vi "FP_Show Hide Items.vi"(8 "Error":errorcluster, 9 "FP Show Hide":T1, 11 "VI":refnum<vi>) -> (0 "Error Out":errorcluster, 3 "VI Out":refnum<vi>)   [LabVIEW 2025]
uses:
  TypeDefs_Utility/Cluster_FP_Show Hide Items.ctl
  TypeDefs_Utility/ENUM_FP_Show-Hide Select.ctl
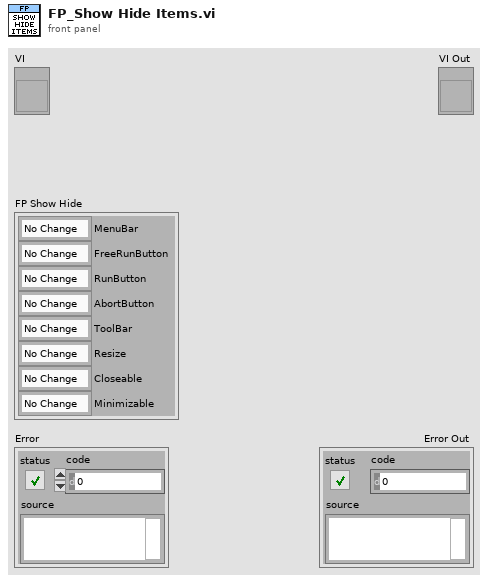
[diagram p1: front panel]
types:
  T1 = typedef "Cluster_FP_Show Hide Items.ctl" = cluster{"MenuBar":T2, "FreeRunButton":T2, "RunButton":T2, "AbortButton":T2, "ToolBar":T2, "Resize":T2, "Closeable":T2, "Minimizable":T2}
  T2 = typedef "ENUM_FP_Show-Hide Select.ctl" = enum16{"No Change", "Hide", "Show"}
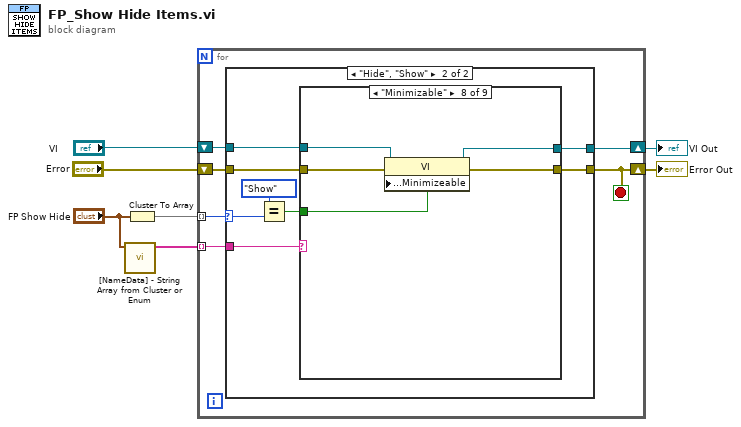
[diagram p0: block diagram]
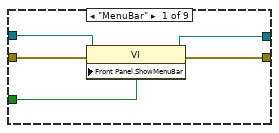
[diagram p3: hidden frame]
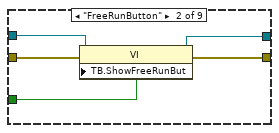
[diagram p4: hidden frame]
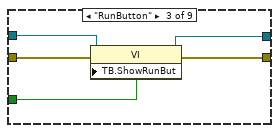
[diagram p5: hidden frame]
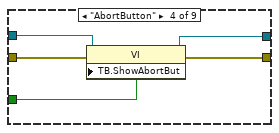
[diagram p6: hidden frame]
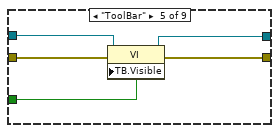
[diagram p7: hidden frame]
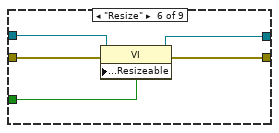
[diagram p8: hidden frame]
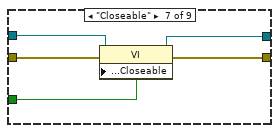
[diagram p9: hidden frame]
diagram:
  n1 = call "[NameData] - String Array from Cluster or Enum.vi"("Enum or\nCluster"="FP Show Hide") -> ("Name Array Out"=w1:string[])  [unwired: 8 in, 2 out]
  n2 = Cluster To Array(cluster="FP Show Hide") -> (array=w2:T2[])
  n3 = for {
    shift-right: [w13] -> w6
    shift-left: "VI" -> [w12]
    shift-right: [w8] -> w7
    shift-left: "Error" -> [w11]
    tunnel: w2 -> [w9] mode=indexing
    tunnel: w1 -> [w10] mode=indexing
    stop <- w8 stop-if-true
    n4 = case shown="\"Hide\", \"Show\"" w9 {
      selector: w9 -> [_ w18]
      tunnel: [w15 w23] -> w13
      tunnel: w12 -> [w15 w22]
      tunnel: w11 -> [w14 w21]
      tunnel: [w14 w20] -> w8
      tunnel: w10 -> [_ w19]
      frame "No Change" {
      }
      frame "Hide", "Show" {
        n5 = Equal?(x=ENUM_FP_Show-Hide_Select."Show" ("y"), y=w18) -> (x = y?=w16:bool)
        n6 = case shown="\"Minimizable\"" w19 {
          tunnel: [w28 w33 w38 w43 w48 w53 w58 w63 w65] -> w23
          tunnel: w22 -> [w27 w32 w37 w42 w47 w52 w57 w62 w65]
          tunnel: w21 -> [w26 w31 w36 w41 w46 w51 w56 w61 w64]
          tunnel: [w25 w30 w35 w40 w45 w50 w55 w60 w64] -> w20
          tunnel: w16 -> [w24 w29 w34 w39 w44 w49 w54 w59 _]
          frame "MenuBar" {
            n7 = property class="VI"(reference=w27, error in=w26, "Front Panel.ShowMenuBar"=w24) -> (reference out=w28:refnum<vi>, error out=w25:errorcluster)
          }
          frame "FreeRunButton" {
            n8 = property class="VI"(reference=w32, error in=w31, "TB.ShowFreeRunBut"=w29) -> (reference out=w33:refnum<vi>, error out=w30:errorcluster)
          }
          frame "RunButton" {
            n9 = property class="VI"(reference=w37, error in=w36, "TB.ShowRunBut"=w34) -> (reference out=w38:refnum<vi>, error out=w35:errorcluster)
          }
          frame "AbortButton" {
            n10 = property class="VI"(reference=w42, error in=w41, "TB.ShowAbortBut"=w39) -> (reference out=w43:refnum<vi>, error out=w40:errorcluster)
          }
          frame "ToolBar" {
            n11 = property class="VI"(reference=w47, error in=w46, "TB.Visible"=w44) -> (reference out=w48:refnum<vi>, error out=w45:errorcluster)
          }
          frame "Resize" {
            n12 = property class="VI"(reference=w52, error in=w51, "Front Panel.Resizeable"=w49) -> (reference out=w53:refnum<vi>, error out=w50:errorcluster)
          }
          frame "Closeable" {
            n13 = property class="VI"(reference=w57, error in=w56, "Front Panel.Closeable"=w54) -> (reference out=w58:refnum<vi>, error out=w55:errorcluster)
          }
          frame "Minimizable" {
            n14 = property class="VI"(reference=w62, error in=w61, "Front Panel.Minimizeable"=w59) -> (reference out=w63:refnum<vi>, error out=w60:errorcluster)
          }
          frame Default {
          }
        }
      }
    }
  }
  "Error Out" <- w7
  "VI Out" <- w6
